vi "QUnits.vi"(8 "error in (no error)":errorcluster, 11 "VISA resource name":refnum<visa-resource-name>) -> (0 "error out":errorcluster, 1 "Unit Label":string, 2 "Units":u32(ring)=1 items=["W"=1, "dB"=2, "dBm"=3, "REL"=4], 3 "VISA resource name out":refnum<visa-resource-name>)   [LabVIEW 2012, in "Newport 1830-C.lvlib"]
doc: "1=Watts\n2=dB\n3=dBm\n4=REL"
uses:
  Newport 1830-C.lvlib
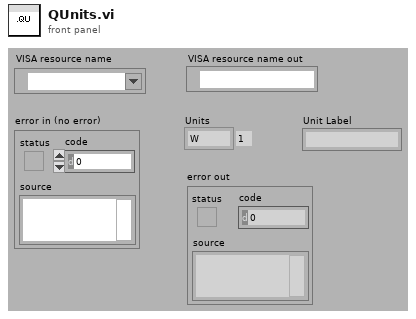
[diagram p1: front panel]
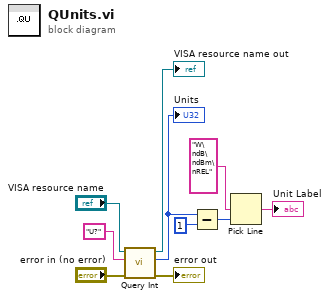
[diagram p0: block diagram]
diagram:
  n1 = call "Query Int.vi"("error in (no error)"="error in (no error)", "write buffer"="U?" ("command"), "VISA resource name In"="VISA resource name") -> ("error out"=→"error out":errorcluster, "int"=w2:u32, "VISA resource name out"=→"VISA resource name out":refnum<visa-resource-name>)  [unwired: 6 in]
  "Units" <- w2
  n2 = Subtract(x=w2, y=u32 1) -> (x-y=w8:u32)
  n3 = Pick Line(multi-line string="W\ndB\ndBm\nREL", line index=w8) -> (output string=→"Unit Label":string)  [unwired: 1 in]
